vi "DSF.Engine.Transceiver.Shutdown.vi"(8 "error in (no error)":errorcluster, 11 "UDP Transceiver in":refnum<class "DSF.Transceiver.UDP.lvclass">) -> (0 "error out":errorcluster, 3 "UDP Transceiver out":refnum<class "DSF.Transceiver.UDP.lvclass">)   [LabVIEW 2017, in "DSF.Transceiver.UDP.lvlib" / "DSF.Transceiver.UDP.lvclass"]
uses:
  DSF.Transceiver.UDP.lvclass
  DSF.Transceiver.UDP.lvclass/DSF.Transceiver.UDP.ctl
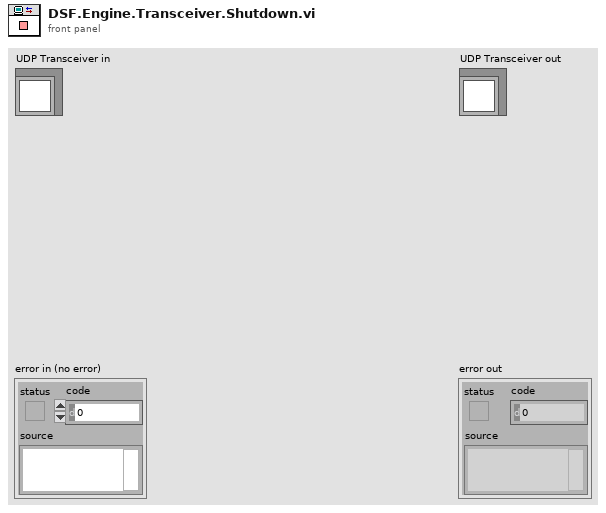
[diagram p1: front panel]
types:
  T1 = typedef "DSF.Transceiver.UDP.lvlib/DSF.Transceiver.UDP.lvclass/DSF.Transceiver.UDP.Tx Parameters.ctl" = cluster{"connection ID":refnum<k16>, "address":u32, "port or service name":u16}
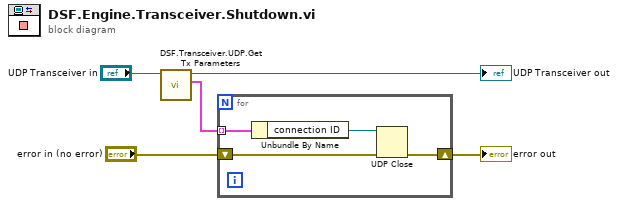
[diagram p0: block diagram]
diagram:
  n1 = call "DSF.Transceiver.UDP.Get Tx Parameters.vi"("DSF.Transceiver.UDP in"="UDP Transceiver in") -> ("Tx parameters"=w2:T1[], "DSF.Transceiver.UDP out"=→"UDP Transceiver out":refnum<class "DSF.Transceiver.UDP.lvclass">)  [unwired: 9 in]
  n2 = for {
    shift-right: [w9] -> w3
    shift-left: "error in (no error)" -> [w8]
    tunnel: w2 -> [w7] mode=indexing
    n3 = Unbundle By Name(w7) -> ("connection ID"=w6:refnum<k16>)
    n4 = UDP Close(connection ID=w6, 8:w8) -> (error out=w9:errorcluster)  [unwired: 1 out]
  }
  "error out" <- w3
